vi "Display.vi"(8 "error in":errorcluster, 11 "Two Button in":refnum<class "Two Button.lvclass">) -> (0 "error out":errorcluster, 3 "Two Button out":refnum<class "Two Button.lvclass">)   [LabVIEW 2021, in "Pop-Up.lvlib" / "Two Button.lvclass"]
doc: "This vi displays the two button popup.\n\n<b>Code Developed By:</b> +\nDaniel Coons +\nhttps://github.com/danielcoons/tsc-pop-up"
uses:
  Two Button.lvclass
  C:/Development/Open Source/tsc-pop-up/Popup/Popup.lvclass
  Two Button.lvclass/Two Button.ctl
  Popup/Popup.lvclass/Popup.ctl
  Popup/Data Member Access/Read Theme.vi
  Theme/Theme.lvclass
  Popup/Popup.lvclass
  user32.dll
panel:
  in  "n-choice":bool
  in  "y-choice":bool
  out "header":bool
  out "2D Picture":picture
  out "String":string
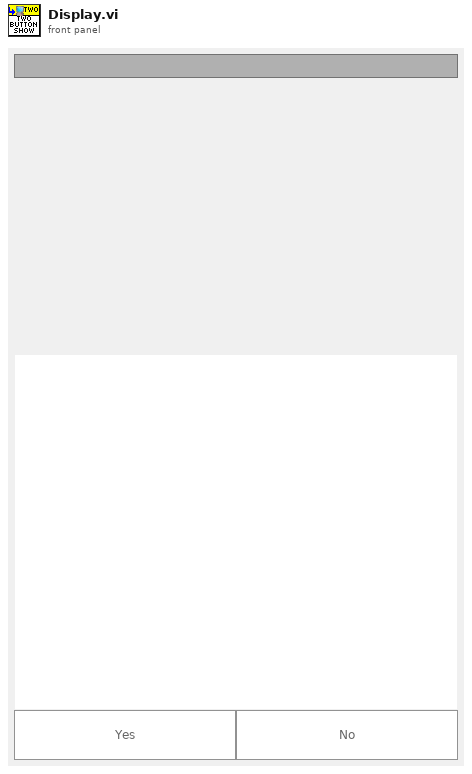
[diagram p1: front panel]
types:
  T1 = typedef "LVPoint32TypeDef.ctl" = cluster{"Horizontal":i32, "Vertical":i32}
  T2 = typedef "LVPositionTypeDef.ctl" = cluster{"Left":i32, "Top":i32}
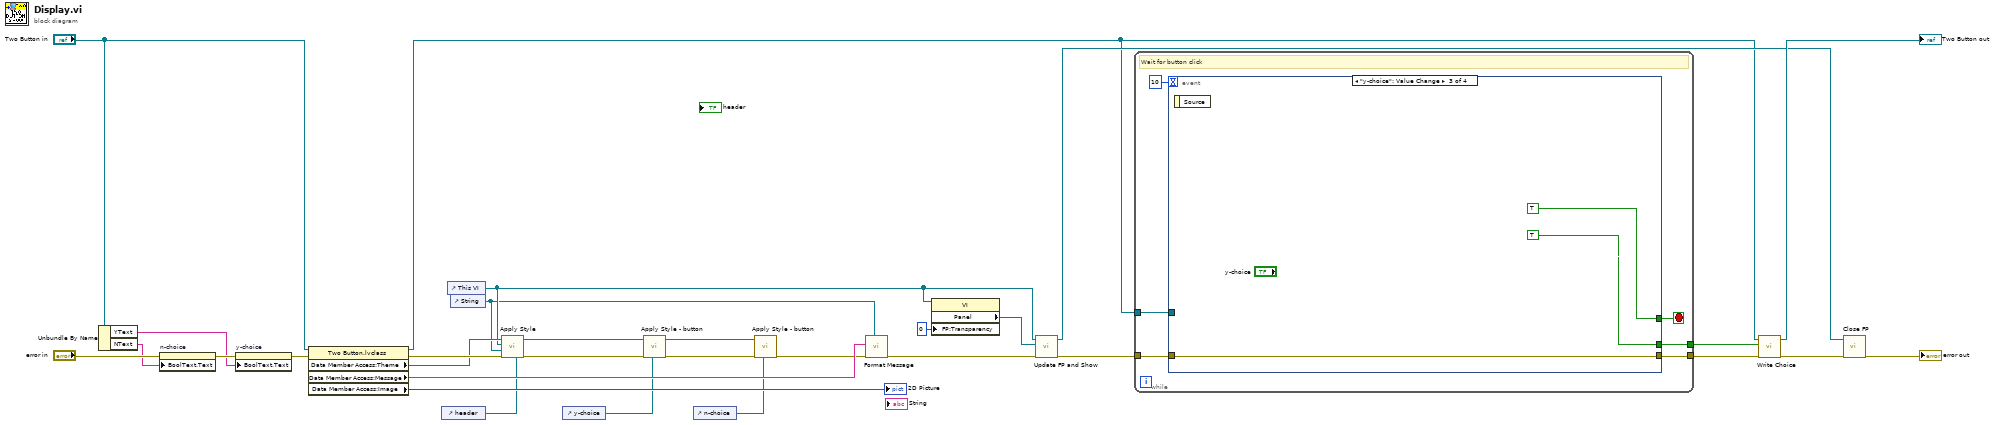
[diagram p0: block diagram]
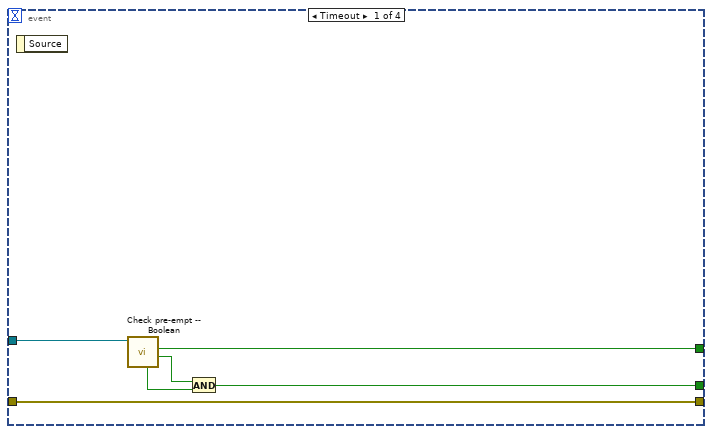
[diagram p2: hidden frame]
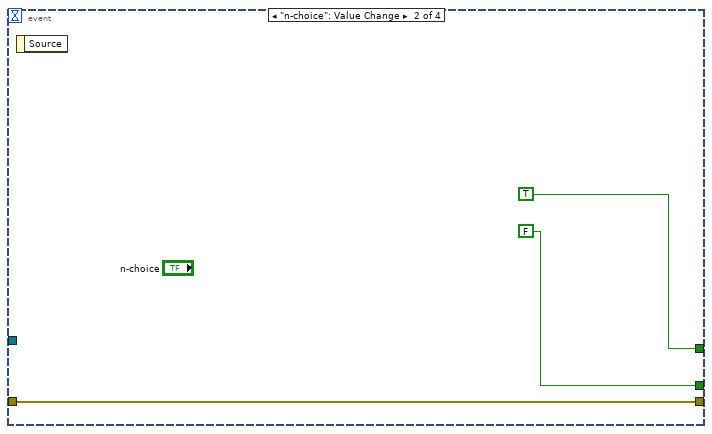
[diagram p3: hidden frame]
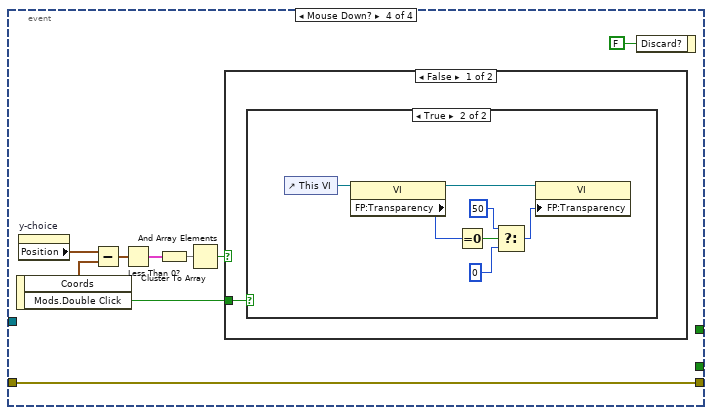
[diagram p4: hidden frame]
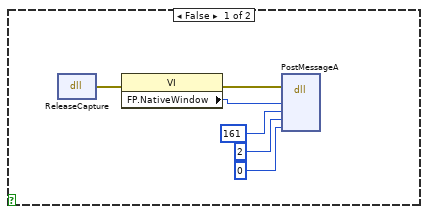
[diagram p5: hidden frame]
diagram:
  n1 = Unbundle By Name("Two Button in") -> ("YText"=w18:string, "NText"=w21:string)
  n2 = property on="n-choice" class="Bool"(error in="error in", "BoolText.Text"=w21) -> (error out=w19:errorcluster)  [unwired: 1 in, 1 out]
  n3 = property on="y-choice" class="Bool"(error in=w19, "BoolText.Text"=w18) -> (error out=w20:errorcluster)  [unwired: 1 in, 1 out]
  n4 = property class="Two Button.lvclass"(reference="Two Button in", error in=w20) -> (reference out=w17:refnum<class "Two Button.lvclass">, error out=w14:errorcluster, "Data Member Access:Theme"=w11:refnum<class "Theme.lvclass">, "Data Member Access:Message"=w15:string, "Data Member Access:Image"=→"2D Picture":picture)
  n5 = control-ref of="header"() -> (w8:refnum<vi>)
  n6 = control-ref of="This VI"() -> (w10:refnum<vi>)
  n7 = control-ref of="String"() -> (w9:refnum<vi>)
  n8 = call "Apply Style.vi"("header ref"=w8, "error in"=w14, "message ref"=w9, "pop up ref"=w10, "Theme in"=w11) -> ("error out"=w12:errorcluster, "Theme out"=w6:refnum<class "Theme.lvclass">)  [unwired: 5 in]
  n9 = control-ref of="y-choice"() -> (w5:refnum<vi>)
  n10 = call "Apply Style - button.vi"("button ref"=w5, "error in"=w12, "Theme in"=w6) -> ("error out"=w7:errorcluster, "Theme out"=w3:refnum<class "Theme.lvclass">)  [unwired: 7 in]
  n11 = control-ref of="n-choice"() -> (w2:refnum<vi>)
  n12 = call "Apply Style - button.vi"("button ref"=w2, "error in"=w7, "Theme in"=w3) -> ("error out"=w4:errorcluster)  [unwired: 7 in, 1 out]
  n13 = call "Format Message.vi"("formatted string"=w9, "error in"=w4, "String Input"=w15) -> ("error out"=w16:errorcluster)  [unwired: 7 in, 1 out]
  n14 = property class="VI"(reference=w10, "FP:Transparency"=u8 0 ("Front Panel Window:Transparency")) -> ("Panel"=w26:refnum<vi>)  [unwired: 1 in, 2 out]
  n15 = call "Update FP and Show.vi"("error in (no error)"=w16, "Panel Ref"=w26, "VI in"=w10) -> ("error out"=w25:errorcluster, "VI out"=w23:refnum<vi>)  [unwired: 7 in]
  n16 = while {
    tunnel: [w36] -> w29
    tunnel: w25 -> [w37]
    tunnel: [w34] -> w28
    tunnel: w17 -> [w33]
    stop <- w35 stop-if-true
    # "Wait for button click"
    n17 = event shown="[2] \"y-choice\": Value Change" {
      selector: _ -> [_ _ _ _]
      dyn-events: _ -> [_ _ _ _]
      timeout: 10 -> [_ _ _ _]
      tunnel: w37 -> [w43 w46 w49 w57]
      tunnel: [w43 w46 w49 w57] -> w36
      tunnel: [w41 TRUE TRUE _] -> w35
      tunnel: [w38 FALSE TRUE _] -> w34
      tunnel: w33 -> [w42 _ _ _]
      event Timeout {
        n18 = event-data() -> ()  [unwired: 1 in, 1 out]
        n19 = call "Check pre-empt -- Boolean.vi"("_Popup in"=w42) -> ("Value?"=w40:bool, "Pre-empted?"=w41:bool, "Type Match?"=w39:bool)  [unwired: 7 in, 1 out]
        n20 = And(x=w40, y=w39) -> (x .and. y?=w38:bool)
      }
      event "n-choice": Value Change {
        n21 = event-data() -> ()  [unwired: 1 in, 1 out]
      }
      event "y-choice": Value Change {
        n22 = event-data() -> ()  [unwired: 1 in, 1 out]
      }
      event Mouse Down? {
        n23 = event-data() -> ("Coords"=w52:T1, "Mods.Double Click"=w50:bool)  [unwired: 1 in]
        n24 = property on="y-choice" class="Bool"() -> ("Position"=w56:T2)  [unwired: 2 in, 2 out]
        n25 = Subtract(x=w56, y=w52) -> (x-y=w55:T2)
        n26 = Less Than 0?(x=w55) -> (x < 0?=w54:cluster{"Left":bool, "Top":bool})
        n27 = Cluster To Array(cluster=w54) -> (array=w53:bool[])
        n28 = And Array Elements(Boolean array=w53) -> (logical AND=w51:bool)
        n29 = case shown="False" w51 {
          tunnel: w50 -> [w59 _]
          frame False {
            n30 = case shown="True" w59 {
              frame False {
                n31 = dll-call lib="user32.dll" fn="ReleaseCapture"() -> (error out=w63:errorcluster)  [unwired: 4 in, 1 out]
                n32 = property class="VI"(error in=w63) -> (error out=w64:errorcluster, "FP.NativeWindow"=w65:u64)  [unwired: 1 in, 1 out]
                n33 = dll-call lib="user32.dll" fn="PostMessageA"(error in=w64, "hWnd"=w65, "Msg"=161, "wParam"=2, "lParam"=0) -> ()  [unwired: 7 in, 2 out]
              }
              frame True {
                n34 = control-ref of="This VI"() -> (w72:refnum<vi>)
                n35 = property class="VI"(reference=w72) -> (reference out=w70:refnum<vi>, "FP:Transparency"=w71:u8)  [unwired: 1 in, 1 out]
                n36 = Equal To 0?(x=w71) -> (x = 0?=w69:bool)
                n37 = Select(t=u8 50, s=w69, f=u8 0) -> (s? t:f=w68:u8)
                n38 = property class="VI"(reference=w70, "FP:Transparency"=w68) -> ()  [unwired: 1 in, 2 out]
              }
            }
          }
          frame True {
          }
        }
        n39 = event-data("Discard?"=FALSE) -> ()  [unwired: 1 in, 1 out]
      }
    }
  }
  n40 = call-dynamic "Write Choice.vi"("error in (no error)"=w29, "Choice"=w28, "_Popup in"=w17) -> ("error out"=w31:errorcluster, "_Popup out"=→"Two Button out":refnum<class "Two Button.lvclass">)  [unwired: 7 in]
  n41 = call "Close FP.vi"("error in (no error)"=w31, "VI in"=w23) -> ("error out"=→"error out":errorcluster)  [unwired: 9 in]
